vi "GetEquipmentAssets.vi"(8 "error in (no error)":errorcluster, 10 "page":i32=1, 11 "service":refnum<class "IcmMessageService.lvclass">) -> (0 "error out":errorcluster, 2 "pages":i32, 3 "AssetNodes":T1[](array[typedef]))   [LabVIEW 2016]
doc: "Queries for all equipment asset nodes, which means they have operating states."
uses:
  <vilib>/addons/InsightCM/MessageBus/MessageLibrary/AssetManager/controls/AssetMgrQueryAssetNodeListRequestBody.ctl
  <vilib>/addons/InsightCM/MessageBus/Base/controls/AssetNodeListQueryParams.ctl
  <vilib>/addons/InsightCM/MessageBus/MessageService/IcmMessageService.lvclass
  <vilib>/addons/InsightCM/MessageBus/Base/controls/AssetState.ctl
  <vilib>/addons/InsightCM/MessageBus/Base/controls/KeyValuePair.ctl
  <vilib>/addons/InsightCM/MessageBus/Base/controls/Metric.ctl
  <vilib>/addons/InsightCM/MessageBus/Base/controls/AssetNodeReference.ctl
  <vilib>/addons/InsightCM/MessageBus/Base/controls/AssetNodeView.ctl
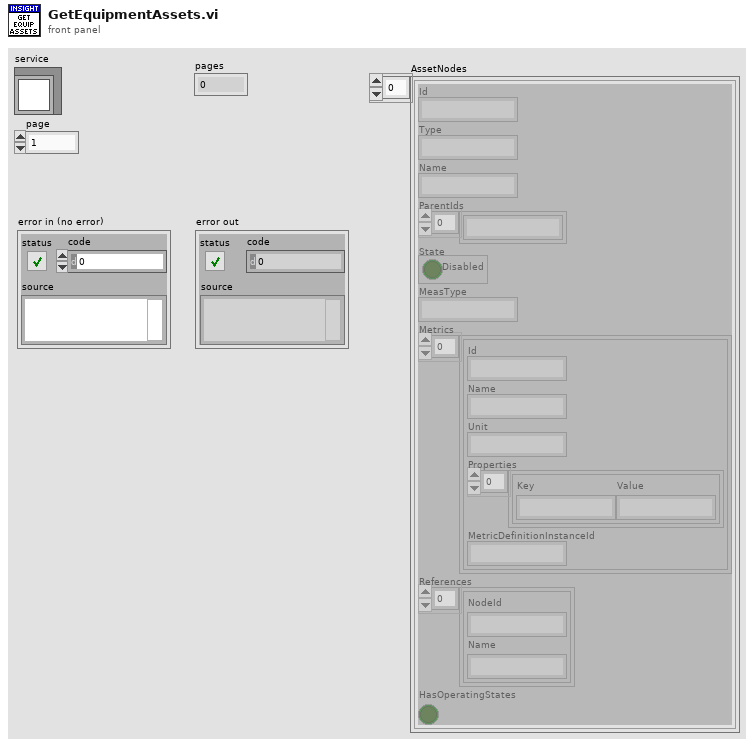
[diagram p1: front panel]
types:
  T1 = typedef "AssetNodeView.ctl" = cluster{"Id":string, "Type":string, "Name":string, "ParentIds":string[], "State":T2, "MeasType":string, "Metrics":T3[], "References":T5[], "HasOperatingStates":bool}
  T2 = typedef "AssetState.ctl" = cluster{"Disabled":bool}
  T3 = typedef "Metric.ctl" = cluster{"Id":string, "Name":string, "Unit":string, "Properties":T4[], "MetricDefinitionInstanceId":string}
  T4 = typedef "KeyValuePair.ctl" = cluster{"Key":string, "Value":string}
  T5 = typedef "AssetNodeReference.ctl" = cluster{"NodeId":string, "Name":string}
  T6 = typedef "AssetMgrQueryAssetNodeListRequestBody.ctl" = cluster{"QueryParams":T7}
  T7 = typedef "AssetNodeListQueryParams.ctl" = cluster{"Type":string, "MeasType":string, "Name":string, "Category":string, "PropKey":string, "PropValue":string, "HasOperatingStates":bool, "NeedsMapping":bool, "HasMetric":string, "Skip":i32, "Take":i32}
  T8 = typedef "Message.ctl" = cluster{"Header":T9, "Body":u8[]}
  T9 = typedef "MessageHeader.ctl" = cluster{"MessageName":string, "Timestamp":i64, "CorrelationId":string, "ContentType":string, "RoutingKey":string, "Properties":T4[]}
  T10 = typedef "AssetMgrQueryAssetNodeListResponseBody.ctl" = cluster{"AssetNodes":T1[], "TotalCount":i32}
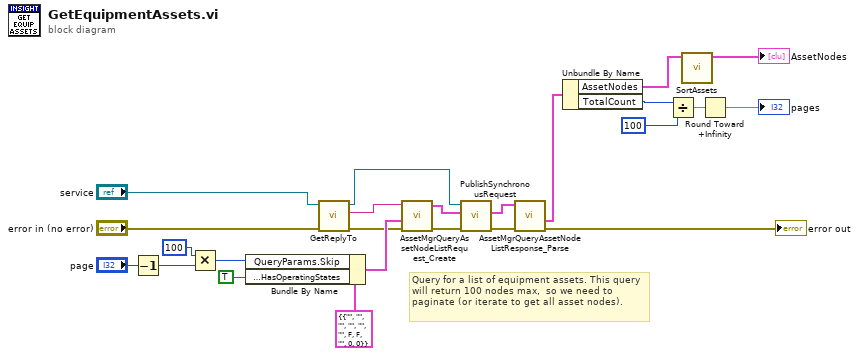
[diagram p0: block diagram]
diagram:
  # "Query for a list of equipment assets. This query will return 100 nodes max,  so we need to paginate (or iterate to get all asset nodes)."
  n1 = Decrement(x="page") -> (x-1=w3:i32)
  n2 = Multiply(x=100, y=w3) -> (x*y=w9:i32)
  n3 = Bundle By Name(cluster=T6 {"QueryParams"={"Type"="", "MeasType"="", "Name"="", "Category"="", "PropKey"="", "PropValue"="", "HasOperatingStates"=FALSE, "NeedsMapping"=FALSE, "HasMetric"="", "Skip"=0, "Take"=0}} ("AssetMgrQueryAssetNodeListRequest"), "QueryParams.Skip"=w9, "QueryParams.HasOperatingStates"=TRUE) -> (w19:T6)
  n4 = call <vilib>:"GetReplyTo.vi"("error in (no error)"="error in (no error)", "service in"="service") -> ("error out"=w16:errorcluster, "reply to"=w14:string, "service out"=w18:refnum<class "IcmMessageService.lvclass">)  [unwired: 7 in]
  n5 = call <vilib>:"AssetMgrQueryAssetNodeListRequest_Create.vi"("error in (no error)"=w16, "AssetMgrQueryAssetNodeListRequest"=w19, "ReplyTo"=w14) -> ("error out"=w17:errorcluster, "Message"=w15:T8)  [unwired: 7 in]
  n6 = call <vilib>:"PublishSynchronousRequest.vi"("error in (no error)"=w17, "request"=w15, "service in"=w18) -> ("error out"=w13:errorcluster, "response"=w12:T8)  [unwired: 6 in, 1 out]
  n7 = call <vilib>:"AssetMgrQueryAssetNodeListResponse_Parse.vi"("error in (no error)"=w13, "Message"=w12) -> ("error out"=→"error out":errorcluster, "Body"=w11:T10)  [unwired: 6 in, 2 out]
  n8 = Unbundle By Name(w11) -> ("AssetNodes"=w2:T1[], "TotalCount"=w7:i32)
  n9 = Divide(x=w7, y=100) -> (x/y=w5:dbl)
  n10 = call "SortAssets.vi"("AssetNodes in"=w2) -> ("AssetNodes out"=→"AssetNodes":T1[])  [unwired: 10 in]
  n11 = Round Toward +Infinity(x=w5) -> (ceil(x): smallest int >= x=→"pages":dbl)
